vi "Execute SQL.vi"(6 "Result?":bool=TRUE, 8 "error in":errorcluster, 10 "SQL":string, 11 "LV-Data.PGSQL":refnum<class "LV-Data.PGSQL.lvclass">) -> (0 "error out":errorcluster, 1 "Result":string[][](array[string]), 2 "SQL out":string, 3 "LV-Data.PGSQL out":refnum<class "LV-Data.PGSQL.lvclass">)   [LabVIEW 2019, in "LV-Data.PGSQL.lvclass"]
uses:
  LV-Data.PGSQL.lvclass
  LV-Data.PGSQL.lvclass/LV-Data.PGSQL.ctl
  <vilib>/JDP Science/PostgreSQL Library/Connection/Execute Command (2D string results).vi
  <vilib>/JDP Science/PostgreSQL Library/Connection/Execute Command (No results).vi
  <vilib>/JDP Science/PostgreSQL Library/Connection/Execute (no results).vi
  <vilib>/JDP Science/PostgreSQL Library/Connection/Execute (Return first result with rows).vi
  <vilib>/JDP Science/PostgreSQL Library/Connection/Execute Single Statement (String Parameters).vi
  <vilib>/JDP Science/PostgreSQL Library/Result/Clear.vi
  <vilib>/JDP Science/PostgreSQL Library/Connection/Execute Command (Result).vi
  <vilib>/JDP Science/PostgreSQL Library/Result/Get all results as 2D strings array.vi
  <vilib>/JDP Science/PostgreSQL Library/Result/Get Column Headers.vi
  <vilib>/JDP Science/PostgreSQL Library/Connection/PQ Connection.lvclass
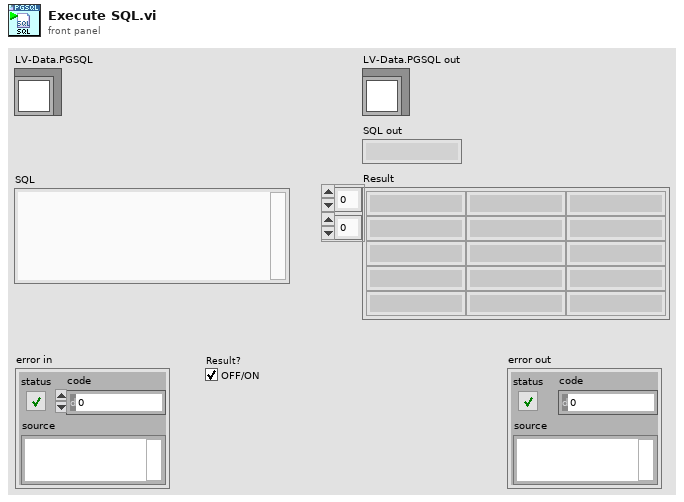
[diagram p1: front panel]
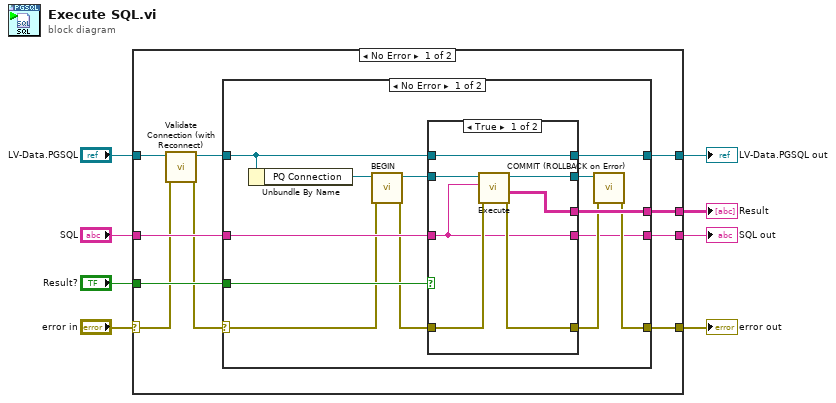
[diagram p0: block diagram]
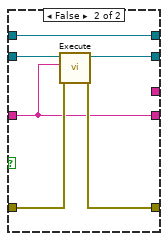
[diagram p2: hidden frame]
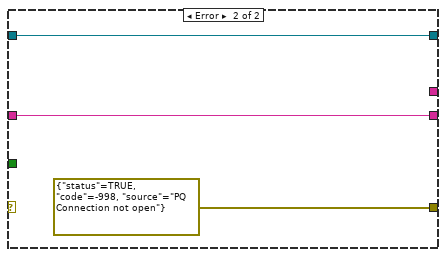
[diagram p3: hidden frame]
diagram:
  n1 = case shown="No Error" "error in" {
    selector: "error in" -> [w10 w49]
    tunnel: [w18 _] -> w8
    tunnel: "SQL" -> [w17 w48]
    tunnel: [w14 w49] -> w6
    tunnel: [w16 w50] -> w5
    tunnel: "LV-Data.PGSQL" -> [w12 w50]
    tunnel: "Result?" -> [w15 _]
    tunnel: [w13 w48] -> w1
    frame No Error {
      n2 = call "Validate Connection (with Reconnect).vi"("error in (no error)"=w10, "LV-Data.PGSQL in"=w12) -> ("error out"=w9:errorcluster, "LV-Data.PGSQL out"=w11:refnum<class "LV-Data.PGSQL.lvclass">)  [unwired: 8 in]
      n3 = case shown="No Error" w9 {
        selector: w9 -> [w25 _]
        tunnel: [w31 _] -> w18
        tunnel: w17 -> [w30 w45]
        tunnel: [w29 w47] -> w16
        tunnel: w11 -> [w20 w47]
        tunnel: w15 -> [w28 _]
        tunnel: [w22 errorcluster {"status"=TRUE, "code"=-998, "source"="PQ Connection not open"} ("error out")] -> w14
        tunnel: [w21 w45] -> w13
        frame No Error {
          n4 = Unbundle By Name(w20) -> ("PQ Connection"=w19:refnum<class "PQ Connection.lvclass">)
          n5 = call <vilib>:"BEGIN.vi"("error in (no error)"=w25, "PQ Connection in"=w19) -> ("error out"=w26:errorcluster, "PQ Connection out"=w27:refnum<class "PQ Connection.lvclass">)  [unwired: 8 in]
          n6 = case shown="True" w28 {
            tunnel: [w38 _] -> w31
            tunnel: w30 -> [w32 w39]
            tunnel: [w36 w43] -> w23
            tunnel: w20 -> [w35 w44]
            tunnel: [w35 w44] -> w29
            tunnel: w26 -> [w37 w42]
            tunnel: w27 -> [w34 w41]
            tunnel: [w33 w40] -> w24
            tunnel: [w32 w39] -> w21
            frame True {
              n7 = call-poly <vilib>:"Execute.vi"("error in (no error)"=w37, "SQL"=w32, "PQ Connection in"=w34) -> ("error out"=w36:errorcluster, "Result"=w38:string[][], "PQ Connection out"=w33:refnum<class "PQ Connection.lvclass">)  [unwired: 4 in, 2 out]
            }
            frame False {
              n8 = call-poly <vilib>:"Execute.vi"("error in (no error)"=w42, "SQL"=w39, "PQ Connection in"=w41) -> ("error out"=w43:errorcluster, "PQ Connection out"=w40:refnum<class "PQ Connection.lvclass">)  [unwired: 7 in]
            }
          }
          n9 = call <vilib>:"COMMIT (ROLLBACK on Error).vi"("error in (no error)"=w23, "PQ Connection in"=w24) -> ("error out"=w22:errorcluster)  [unwired: 8 in, 1 out]
        }
        frame Error {
        }
      }
    }
    frame Error {
    }
  }
  "Result" <- w8
  "error out" <- w6
  "LV-Data.PGSQL out" <- w5
  "SQL out" <- w1
